vi "Set Motor Speed.vi"(7 "Max Velocity":dbl, 11 "Front Left":T1 {"Angle" scale format="%.3f"; "Velocity" scale=-1.0..1.0 scale format="%.1f"}) -> (3 "Velocity Value Set Out":dbl)   [LabVIEW 2023, in "TShirtWork-SwerveDrive_ACT_ts.lvlib"]
uses:
  TShirtWork-SwerveDrive_ACT_ts.lvlib
  Shared Code/TypeDefs/Level_Velocity plus-minus 1.ctl
  Shared Code/TypeDefs/Dial_Compase heading unit circle CCW positive.ctl
  Shared Code/TypeDefs/Cluster_Module Velocity-Direction-Rotations.ctl
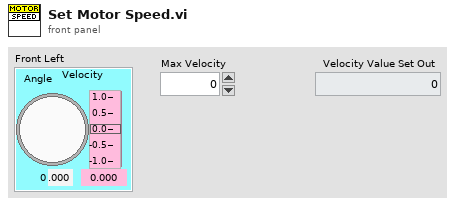
[diagram p1: front panel]
types:
  T1 = typedef "Cluster_Module Velocity-Direction-Rotations.ctl" = cluster{"Velocity":T2, "Angle":T3, "Rotations Count":dbl}
  T2 = typedef "Level_Velocity plus-minus 1.ctl" = dbl
  T3 = typedef "Dial_Compase heading unit circle CCW positive.ctl" = dbl
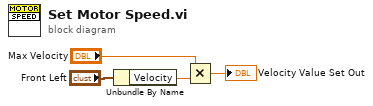
[diagram p0: block diagram]
diagram:
  n1 = Unbundle By Name("Front Left") -> ("Velocity"=w2:T2)
  n2 = Multiply(x="Max Velocity", y=w2) -> (x*y=→"Velocity Value Set Out":T2)
